vi "Send Current.vi"(8 "error in":errorcluster, 11 "69X_79X in":refnum<class "69X_79X.lvclass">) -> (0 "error out":errorcluster, 3 "69X_79X out":refnum<class "69X_79X.lvclass">)   [LabVIEW 2019, in "69X_79X.lvlib" / "69X_79X.lvclass"]
uses:
  Library/69X_79X.lvclass
  C:/Users/Public/Documents/Development/builds/Instruments/PowerSupply.lvlibp/Library/PowerSupply.lvclass
  Accessors/Read Local Resource.vi
  Accessors/Write Local Resource.vi
  <instrlib>/Agilent N6900 N7900 Series/Agilent N6900 N7900 Series.lvlib
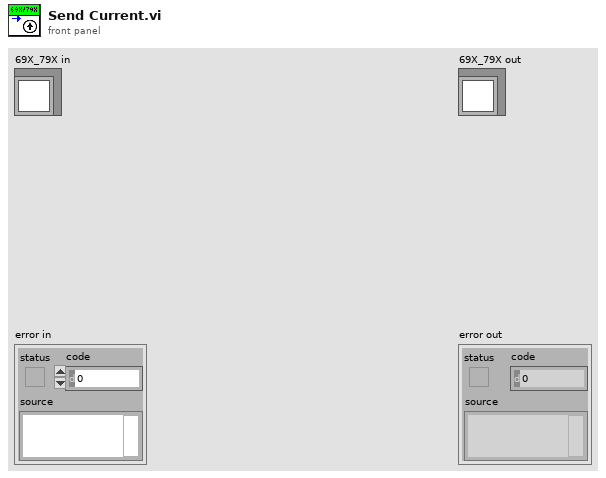
[diagram p1: front panel]
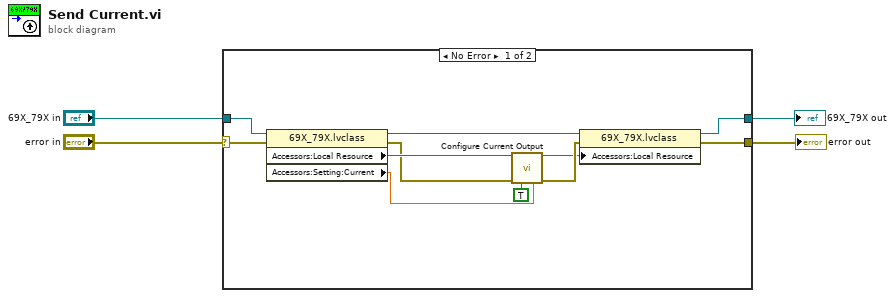
[diagram p0: block diagram]
diagram:
  n1 = case shown="No Error" "error in" {
    selector: "error in" -> [w13 w16]
    tunnel: "69X_79X in" -> [w14 w17]
    tunnel: [w9 w17] -> w4
    tunnel: [w10 w16] -> w3
    frame No Error {
      n2 = property class="69X_79X.lvclass"(reference=w14, error in=w13) -> (reference out=w11:refnum<class "69X_79X.lvclass">, error out=w6:errorcluster, "Accessors:Local Resource"=w7:refnum<visa-resource-name>, "Accessors:Setting:Current"=w5:dbl)
      n3 = call <instrlib>:"Configure Current Output.vi"("VISA resource name"=w7, "error in (no error)"=w6, "Enable Voltage Priority (False)"=TRUE, "Voltage Priority Current Upper Limit (2.50A)"=w5) -> ("VISA resource name out"=w12:refnum<visa-resource-name>, "error out"=w15:errorcluster)  [unwired: 10 in]
      n4 = property class="69X_79X.lvclass"(reference=w11, error in=w15, "Accessors:Local Resource"=w12) -> (reference out=w9:refnum<class "69X_79X.lvclass">, error out=w10:errorcluster)
    }
    frame Error {
    }
  }
  "error out" <- w3
  "69X_79X out" <- w4
